vi "Localisation_To_Graph(SubVI).vi"(6 "Current_Position_out":T1, 7 "Refnum in":refnum<k20>, 8 "Y_Arr":sgl[](array[numeric]), 9 "X_arr":sgl[](array[numeric]), 10 "Est_Y_arr":dbl[](array[numeric]), 11 "Est_X_arr":dbl[](array[numeric])) -> (0 "Y_arr_out":sgl[](array[numeric]), 1 "X_Arr_out":sgl[](array[numeric]), 2 "Est_Y_arr_out":dbl[](array[numeric]), 3 "Est_X_Arr_out":dbl[](array[numeric]), 4 "Array":cluster{dbl[], dbl[]}[](array[cluster]), 5 "Refnum out":refnum<k20>)   [LabVIEW 2017]
doc: "Display robot's path and current position in a graph"
uses:
  Ctl/Current_Position.ctl
  <resource>/objmgr/LVODE.rc
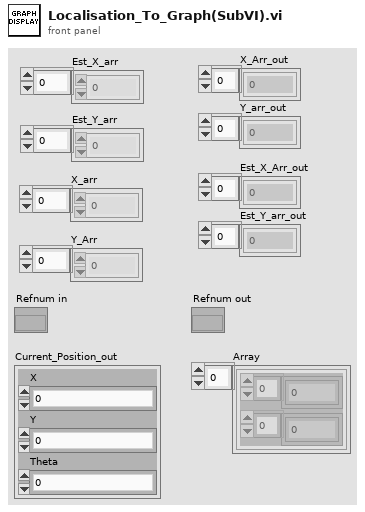
[diagram p1: front panel]
types:
  T1 = typedef "Current_Position.ctl" = cluster{"X":dbl, "Y":dbl, "Theta":dbl}
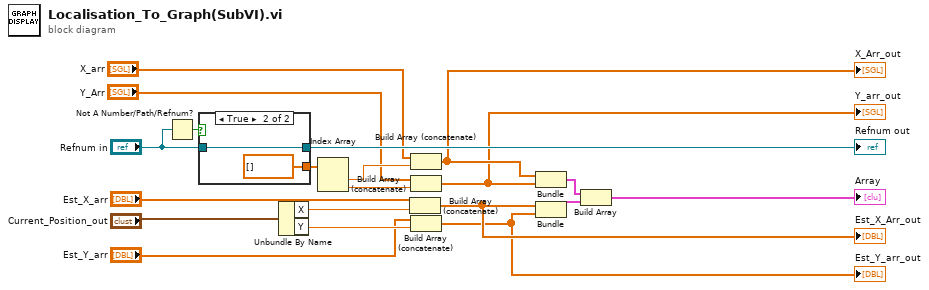
[diagram p0: block diagram]
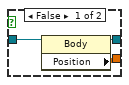
[diagram p2: hidden frame]
diagram:
  n1 = Not A Number/Path/Refnum?(number/path/refnum="Refnum in") -> (NaN/Path/Refnum?=w2:bool)
  n2 = case shown="True" w2 {
    tunnel: [w23 w25] -> w20
    tunnel: [w22 sgl[] [] ("Position")] -> w13
    tunnel: "Refnum in" -> [w21 w25]
    frame False {
      n3 = property class="Body"(reference=w21) -> (reference out=w23:refnum<k20>, "Position"=w22:sgl[])  [unwired: 1 in, 1 out]
    }
    frame True {
    }
  }
  "Refnum out" <- w20
  n4 = Unbundle By Name("Current_Position_out") -> ("X"=w15:dbl, "Y"=w16:dbl)
  n5 = Index Array(array=w13) -> (element #1=w11:sgl, element #2=w12:sgl)  [unwired: 2 in]
  n6 = Build Array (concatenate)("Est_X_arr", w15) -> (w9:dbl[])
  "Est_X_Arr_out" <- w9
  n7 = Build Array (concatenate)("X_arr", w11) -> (w10:sgl[])
  "X_Arr_out" <- w10
  n8 = Build Array (concatenate)("Y_Arr", w12) -> (w3:sgl[])
  "Y_arr_out" <- w3
  n9 = Build Array (concatenate)("Est_Y_arr", w16) -> (w8:dbl[])
  "Est_Y_arr_out" <- w8
  n10 = Bundle(w10, w3) -> (w17:cluster{sgl[], sgl[]})  [unwired: 1 in]
  n11 = Bundle(w9, w8) -> (w18:cluster{dbl[], dbl[]})  [unwired: 1 in]
  n12 = Build Array(w17, w18) -> (→"Array":cluster{dbl[], dbl[]}[])
